vi "国际象棋单人.vi"() -> ()   [LabVIEW 2017]
panel:
  in  "数值":u8
  out "过程信息":string[](array[string])
  in  "新游戏":bool
  in  "Buttons":bool[][](array[boolean])=[[FALSE, FALSE, FALSE, FALSE, FALSE, FALSE, FALSE, FALSE], [FALSE, FALSE, FALSE, FALSE, FALSE, FALSE, FALSE, FALSE], [FALSE, FALSE, FALSE, FALSE, FALSE, FALSE, FALSE, FALSE], [FALSE, FALSE, FALSE, FALSE, FALSE, FALSE, FALSE, FALSE], [FALSE, FALSE, FALSE, FALSE, FALSE, FALSE, FALSE, FALSE], [FALSE, FALSE, FALSE, FALSE, FALSE, FALSE, FALSE, FALSE], [FALSE, FALSE, FALSE, FALSE, FALSE, FALSE, FALSE, FALSE], [FALSE, FALSE, FALSE, FALSE, FALSE, FALSE, FALSE, FALSE]]
  out "Indicator":bool[][](array[boolean])
  out "Y":i32
  out "X":i32
  in  "停止":bool
  out "移动方":enum16{"银色", "黑色"}(ring)
  out "棋盘":T1
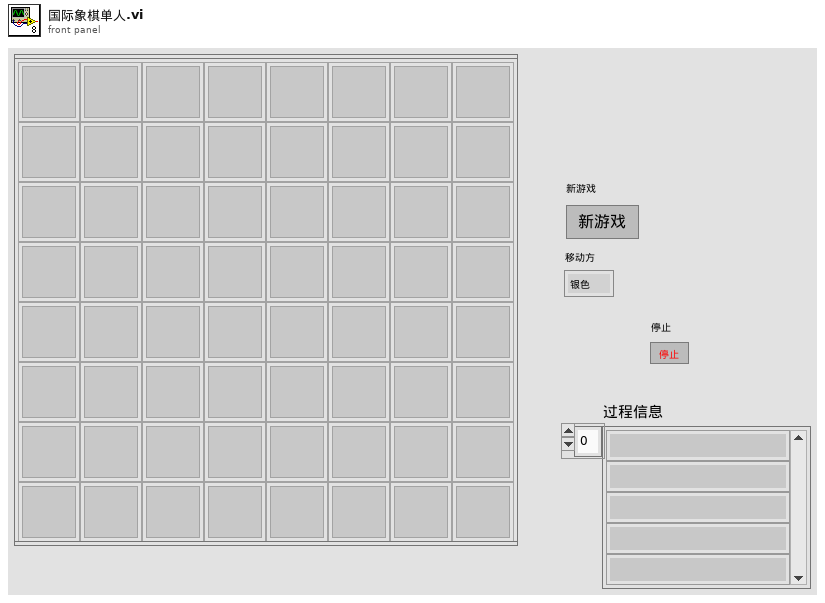
[diagram p1: front panel]
types:
  T1 = typedef "棋盘.ctl" = u16[][]
  T2 = cluster{"棋盘":u16[][], "银色棋子":cluster{"棋子类型":enum16{"士兵", "骑士", "主教", "战车", "皇后", "国王", "空"}, "X":u8, "Y":u8}[], "黑色棋子":cluster{"棋子类型":enum16{"士兵", "骑士", "主教", "战车", "皇后", "国王", "空"}, "X":u8, "Y":u8}[], "移动方":enum16{"银色", "黑色"}}
  T3 = cluster{"棋盘":u16[][], "银色棋子":cluster{"棋子类型":enum16{"士兵", "骑士", "主教", "战车", "皇后", "国王", "空"}, "X":u8, "Y":u8}[], "黑色棋子":cluster{"棋子类型":enum16{"士兵", "骑士", "主教", "战车", "皇后", "国王", "空"}, "X":u8, "Y":u8}[], "移动方":enum16{"银色", "黑色"}}[]
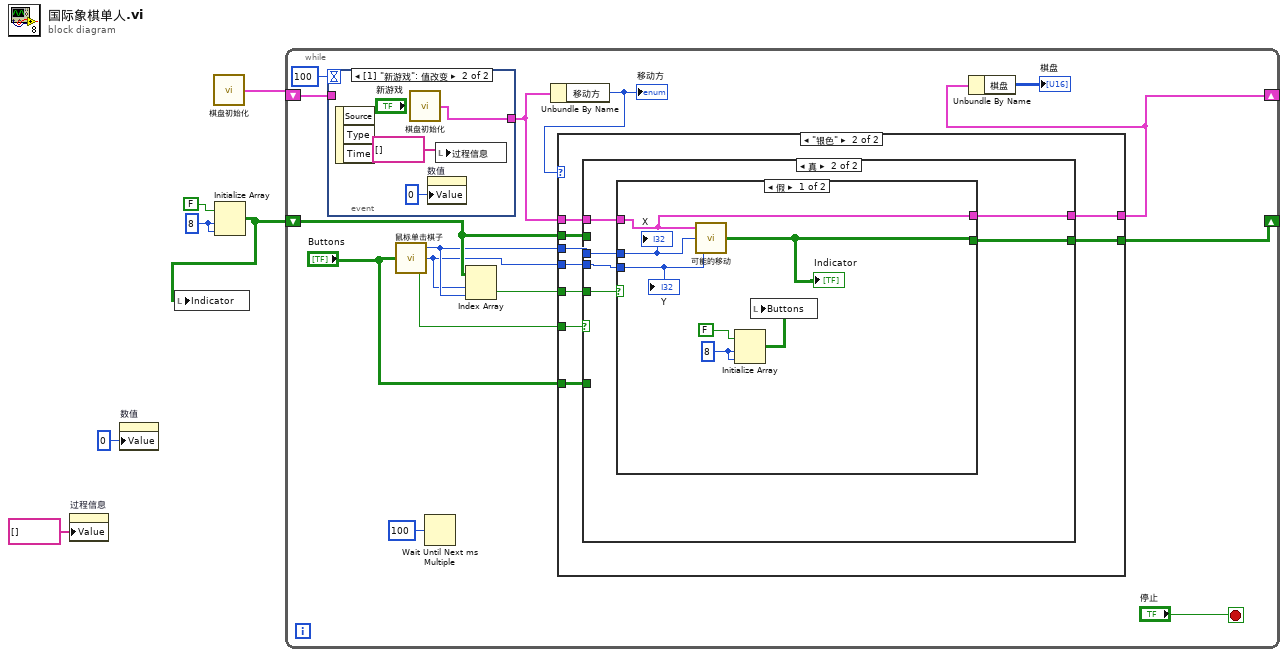
[diagram p0: block diagram]
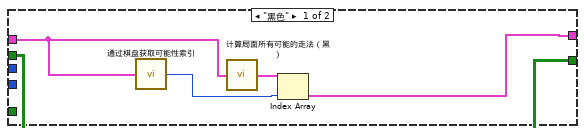
[diagram p2: hidden frame]
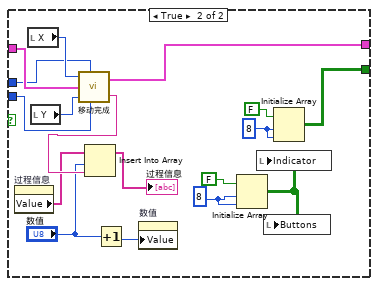
[diagram p4: hidden frame]
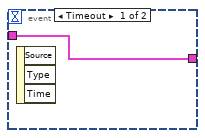
[diagram p5: hidden frame]
diagram:
  w5 = 8 ("维数大小")
  n1 = property on="过程信息" class="Arr (严格)"("Value"=string[] [] ("过程信息")) -> ()  [unwired: 2 in, 2 out]
  n2 = property on="数值" class="DigNum (严格)"("Value"=u8 0 ("数值")) -> ()  [unwired: 2 in, 2 out]
  n3 = call "棋盘初始化.vi"() -> ("游戏"=w6:T2)
  n4 = Initialize Array(FALSE, w5, w5) -> (w3:bool[][])
  n5 = local write "Indicator"(w3) -> ()
  n6 = while {
    shift-right: [w16] -> _
    shift-left: w6 -> [w11]
    shift-right: [w8] -> _
    shift-left: w3 -> [w21]
    stop <- "停止" stop-if-true
    n7 = event shown="[1] \"新游戏\": 值改变" {
      selector: _ -> [_ _]
      dyn-events: _ -> [_ _]
      timeout: 100 -> [_ _]
      tunnel: [w68 w71] -> w12
      tunnel: w11 -> [w68 _]
      event Timeout {
        n8 = event-data() -> ()  [unwired: 1 in, 3 out]
      }
      event "新游戏": Value Change {
        n9 = event-data() -> ()  [unwired: 1 in, 3 out]
        n10 = call "棋盘初始化.vi"() -> ("游戏"=w71:T2)
        n11 = property on="数值" class="DigNum (严格)"("Value"=u8 0 ("数值")) -> ()  [unwired: 2 in, 2 out]
        n12 = local write "过程信息"(string[] [] ("数组")) -> ()
      }
    }
    n13 = call "鼠标单击棋子.vi"("按钮"="Buttons") -> ("X"=w20:i32, "Y"=w19:i32, "是否单击"=w18:bool)
    n14 = Wait Until Next ms Multiple(millisecond multiple=u32 100 ("毫秒倍数")) -> ()  [unwired: 1 out]
    n15 = Index Array(array=w21, index (row)=w19, index (col)=w20) -> (element=w17:bool)
    n16 = Unbundle By Name(w12) -> ("移动方"=w7:enum16{"银色", "黑色"})
    "移动方" <- w7
    n17 = case shown="\"银色\"" w7 {
      tunnel: w21 -> [w22 w35]
      tunnel: w20 -> [_ w34]
      tunnel: w19 -> [_ w33]
      tunnel: w18 -> [_ w32]
      tunnel: w17 -> [_ w31]
      tunnel: [w23 w30] -> w16
      tunnel: "Buttons" -> [_ w29]
      tunnel: w12 -> [w26 w28]
      tunnel: [w22 w27] -> w8
      frame "黑色" {
        n18 = call "通过棋盘获取可能性索引.vi"("输入的棋盘"=w26) -> ("索引"=w24:i32)
        n19 = call "计算局面所有可能的走法（黑）.vi"("输入的棋盘"=w26) -> ("可能移动"=w25:T3)
        n20 = Index Array(array=w25, index=w24) -> (element=w23:T2)
      }
      frame "银色" {
        n21 = case shown="真" w32 {
          tunnel: w28 -> [w36 w40]
          tunnel: w35 -> [w37 _]
          tunnel: w34 -> [_ w43]
          tunnel: w33 -> [_ w42]
          tunnel: w31 -> [_ w41]
          tunnel: w29 -> [_ _]
          tunnel: [w36 w39] -> w30
          tunnel: [w37 w38] -> w27
          frame False {
          }
          frame True {
            n22 = case shown="假" w41 {
              tunnel: w43 -> [w50 w58]
              tunnel: w42 -> [w49 w57]
              tunnel: w40 -> [w46 w67]
              tunnel: [w46 w56] -> w39
              tunnel: [w44 w64] -> w38
              frame False {
                w48 = 8 ("维数大小")
                n23 = call "可能的移动.vi"("Y"=w49, "X"=w50, "游戏"=w46) -> ("输出数组"=w44:bool[][])
                "Indicator" <- w44
                n24 = Initialize Array(FALSE, w48, w48) -> (w45:bool[][])
                n25 = local write "Buttons"(w45) -> ()
                "X" <- w50
                "Y" <- w49
              }
              frame True {
                w62 = 8 ("维数大小")
                w65 = 8 ("维数大小")
                n26 = property on="过程信息" class="Arr (严格)"() -> ("Value"=w51:string[])  [unwired: 2 in, 2 out]
                n27 = local read "X"() -> (w60:i32)
                n28 = local read "Y"() -> (w59:i32)
                n29 = call "移动完成.vi"("原始X"=w60, "移动后的X"=w58, "输入的棋盘"=w67, "原始Y"=w59, "移动后的Y"=w57) -> ("输出的棋盘"=w56:T2, "结果"=w55:string)
                n30 = Insert Into Array(array=w51, index="数值", new element=w55) -> (→"过程信息":string[])
                n31 = Increment(x="数值") -> (x+1=w53:u8)
                n32 = property on="数值" class="DigNum (严格)"("Value"=w53) -> ()  [unwired: 2 in, 2 out]
                n33 = Initialize Array(FALSE, w62, w62) -> (w61:bool[][])
                n34 = local write "Indicator"(w61) -> ()
                n35 = local write "Buttons"(w61) -> ()
                n36 = Initialize Array(FALSE, w65, w65) -> (w64:bool[][])
              }
            }
          }
        }
      }
    }
    n37 = Unbundle By Name(w16) -> ("棋盘"=→"棋盘":u16[][])
  }
